vi "4155C Config V Stress v2.0.vi"(1 "Display on/off":bool, 2 "Stress V - Gate":u32(ring)=2 items=["SMU1  ", "SMU2  ", "SMU3  ", "SMU4  ", "SMU5  ", "SMU6  "], 4 "Stress V - Drain":u32(ring)=1 items=["SMU1  ", "SMU2  ", "SMU3  ", "SMU4  ", "SMU5  ", "SMU6  "], 5 "Stress V - Source/Common":u32(ring) items=["SMU1  ", "SMU2  ", "SMU3  ", "SMU4  ", "SMU5  ", "SMU6  "], 6 "IG compliance":dbl min=0.0 max=100000000000.0 format="%.15e", 7 "ID compliance":dbl min=0.0 max=100000000000.0 format="%.15e", 8 "error in (no error)":errorcluster, 9 "VG":dbl min=0.0 max=100000000000.0 format="%.15e", 10 "VD":dbl min=0.0 max=100000000000.0 format="%.15e", 11 "VISA session":refnum<visa-resource-name>) -> (0 "error out":errorcluster, 3 "dup VISA resource name":refnum<visa-resource-name>)   [LabVIEW 2016]
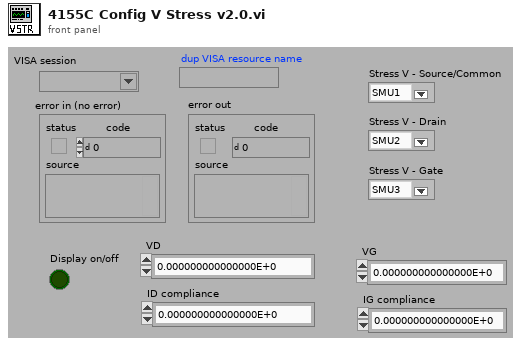
[diagram p1: front panel]
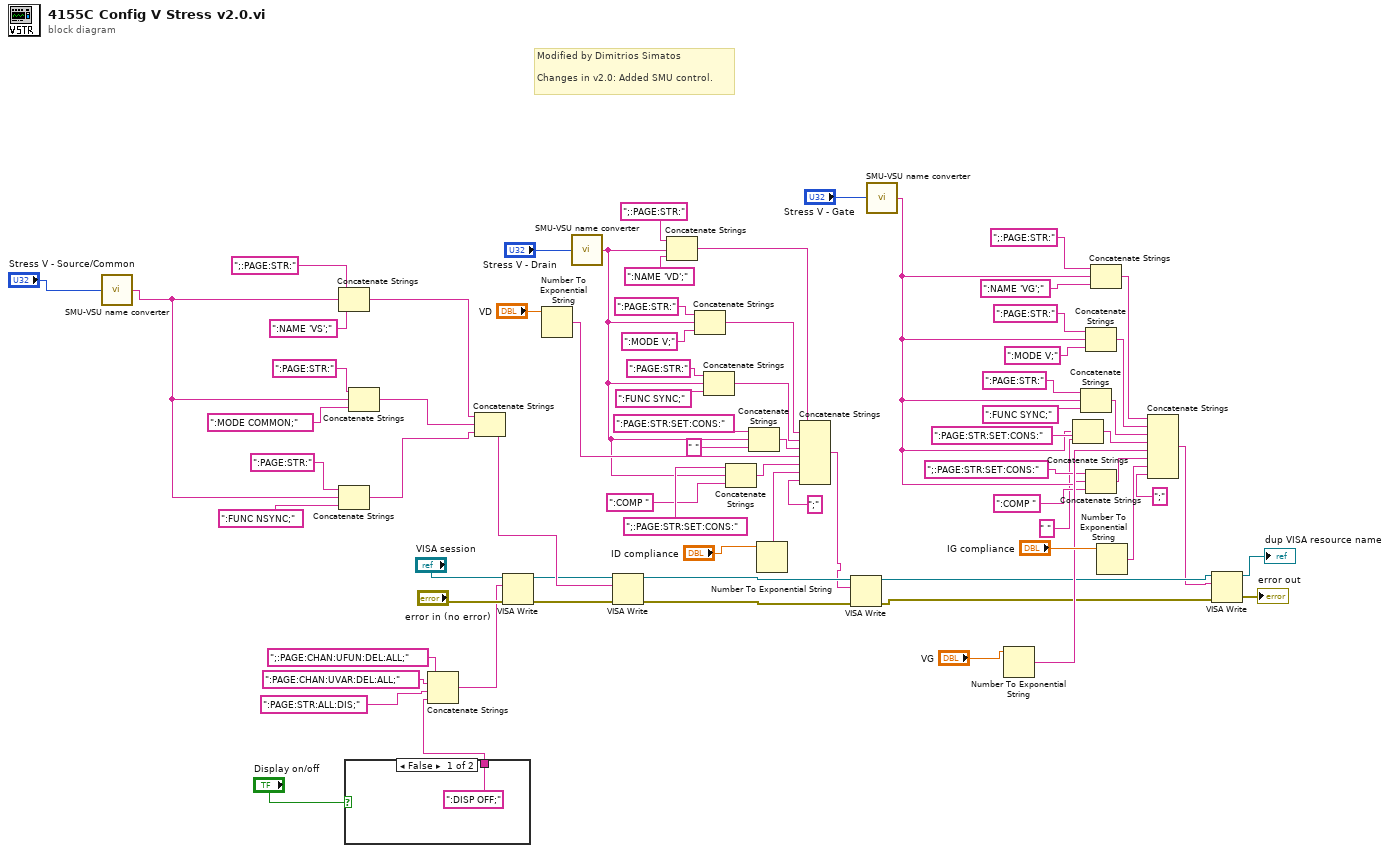
[diagram p0: block diagram]
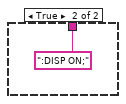
[diagram p2: hidden frame]
diagram:
  # "Modified by Dimitrios Simatos\n\nChanges in v2.0: Added SMU control."
  n1 = call "SMU-VSU name converter.vi"("unit to configure"="Stress V - Source/Common") -> ("SMU/VSU to be configured"=w43:string)
  n2 = Concatenate Strings(";:PAGE:STR:", w43, ":NAME 'VS';") -> (w42:string)
  n3 = Concatenate Strings(":PAGE:STR:", w43, ":FUNC NSYNC;") -> (w40:string)
  n4 = case shown="False" "Display on/off" {
    tunnel: [":DISP OFF;" ("write buffer (\"\")") ":DISP ON;" ("write buffer (\"\")")] -> w68
    frame False {
    }
    frame True {
    }
  }
  n5 = Concatenate Strings(":PAGE:STR:", w43, ":MODE COMMON;") -> (w41:string)
  n6 = Concatenate Strings(";:PAGE:CHAN:UFUN:DEL:ALL;", ":PAGE:CHAN:UVAR:DEL:ALL;", ":PAGE:STR:ALL:DIS;", w68) -> (w69:string)
  n7 = Concatenate Strings(w42, w41, w40) -> (w54:string)
  n8 = VISA Write(VISA resource name="VISA session", write buffer=w69, error in (no error)="error in (no error)") -> (VISA resource name out=w53:refnum<visa-resource-name>, error out=w52:errorcluster)  [unwired: 1 out]
  n9 = Number To Exponential String(number="VD") -> (E-format string=w62:string)  [unwired: 3 in]
  n10 = call "SMU-VSU name converter.vi"("unit to configure"="Stress V - Drain") -> ("SMU/VSU to be configured"=w19:string)
  n11 = VISA Write(VISA resource name=w53, write buffer=w54, error in (no error)=w52) -> (VISA resource name out=w74:refnum<visa-resource-name>, error out=w73:errorcluster)  [unwired: 1 out]
  n12 = Concatenate Strings(";:PAGE:STR:", w19, ":NAME 'VD';") -> (w30:string)
  n13 = Concatenate Strings(":PAGE:STR:", w19, ":MODE V;") -> (w27:string)
  n14 = Concatenate Strings(":PAGE:STR:", w19, ":FUNC SYNC;") -> (w24:string)
  n15 = Concatenate Strings(";:PAGE:STR:SET:CONS:", w19, ":COMP ") -> (w18:string)
  n16 = Concatenate Strings(":PAGE:STR:SET:CONS:", w19, " " ("string")) -> (w22:string)
  n17 = Number To Exponential String(number="ID compliance") -> (E-format string=w60:string)  [unwired: 3 in]
  n18 = Concatenate Strings(w30, w27, w24, w22, w62, w18, w60, ";" ("Substring")) -> (w51:string)
  n19 = VISA Write(VISA resource name=w74, write buffer=w51, error in (no error)=w73) -> (VISA resource name out=w49:refnum<visa-resource-name>, error out=w50:errorcluster)  [unwired: 1 out]
  n20 = call "SMU-VSU name converter.vi"("unit to configure"="Stress V - Gate") -> ("SMU/VSU to be configured"=w3:string)
  n21 = Number To Exponential String(number="VG") -> (E-format string=w57:string)  [unwired: 3 in]
  n22 = Concatenate Strings(":PAGE:STR:SET:CONS:", w3, " " ("string")) -> (w7:string)
  n23 = Concatenate Strings(":PAGE:STR:", w3, ":FUNC SYNC;") -> (w11:string)
  n24 = Concatenate Strings(":PAGE:STR:", w3, ":MODE V;") -> (w14:string)
  n25 = Concatenate Strings(";:PAGE:STR:SET:CONS:", w3, ":COMP ") -> (w6:string)
  n26 = Concatenate Strings(";:PAGE:STR:", w3, ":NAME 'VG';") -> (w15:string)
  n27 = Number To Exponential String(number="IG compliance") -> (E-format string=w55:string)  [unwired: 3 in]
  n28 = Concatenate Strings(w15, w14, w11, w7, w57, w6, w55, ";" ("Substring")) -> (w48:string)
  n29 = VISA Write(VISA resource name=w49, write buffer=w48, error in (no error)=w50) -> (VISA resource name out=→"dup VISA resource name":refnum<visa-resource-name>, error out=→"error out":errorcluster)  [unwired: 1 out]
